vi "CC FITS Write DEC Header.vi"(10 "Detector #":u16, 11 "HK Channel":refnum<class "HK Table.lvclass">) -> (1 "ROT out":dbl, 2 "DEC out":dbl, 3 "RA out":dbl)   [LabVIEW 2024]
uses:
  hk-channel-class/hk-channel-class/HK Table/HK Table.lvclass
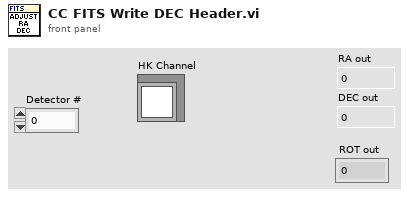
[diagram p1: front panel]
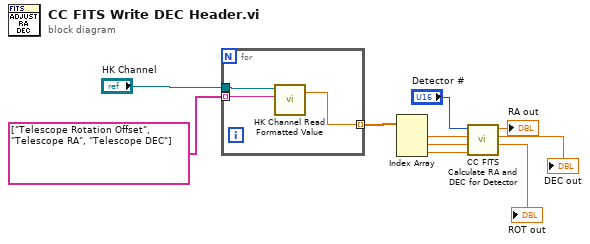
[diagram p0: block diagram]
diagram:
  n1 = for {
    tunnel: string[] ["Telescope Rotation Offset", "Telescope RA", "Telescope DEC"] -> [w13] mode=indexing
    tunnel: "HK Channel" -> [w12]
    tunnel: [w11] -> w8 mode=indexing
    n2 = call-dynamic "HK Channel Read Formatted Value.vi"("Name"=w13, "HK Table.lvclass"=w12) -> ("Value"=w11:dbl)  [unwired: 2 in, 7 out]
  }
  n3 = Index Array(array=w8) -> (element #1=w7:dbl, element #2=w5:dbl, element #3=w4:dbl)  [unwired: 3 in]
  n4 = call "CC FITS Calculate RA and DEC for Detector.vi"("DEC"=w4, "RA"=w5, "ROT"=w7, "Detector #"="Detector #") -> ("ROT out"=→"ROT out":dbl, "DEC out"=→"DEC out":dbl, "RA out"=→"RA out":dbl)  [unwired: 4 in, 1 out]
